vi "Cross_Moments.vi"(0 "U":dbl[](array[numeric]) format="%.2f", 1 "W":dbl[](array[numeric]) format="%.2f", 2 "Block No":i32=1, 3 "Inst names":string[](array[string]), 5 "Shift in":dbl[](array[numeric]) format="%.2f", 8 "Indicies":i32[](array[numeric])) -> (14 "Correlations Only":string[](array[string]), 15 "All Results for file":string[](array[string]), 17 "Velocity Cluster Array Out":T1[](array[typedef]) {"u^4" format="%.2f"; "Mean % Err" format="%.2f"; "u^4/(u^2)^2 -3" format="%.2f"; "u^3/(u^2)^(1.5)" format="%.2f"; "u^2" format="%.2f"; "% u'/U" format="%.2f"; "U" format="%.2f"}, 19 "Shift out":dbl[](array[numeric]) format="%.2f")   [LabVIEW 2010]
uses:
  Controls/Velocity_cluster.ctl
  Globals/Meas_global.vi
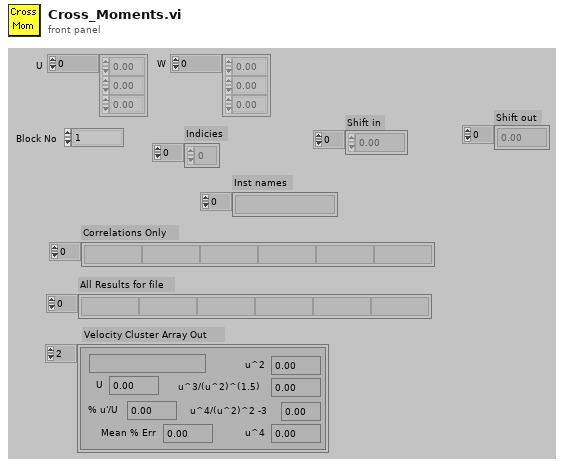
[diagram p1: front panel]
types:
  T1 = typedef "Velocity_cluster.ctl" = cluster{"Name":string, "U":dbl, "u^2":dbl, "u^3/(u^2)^(1.5)":dbl, "u^4/(u^2)^2 -3":dbl, "% u'/U":dbl, "Mean % Err":dbl, "u^4":dbl}
  T2 = typedef "Correlation_cluster.ctl" = cluster{"U inst":string, "W inst":string, "uw":dbl, "uw/u'w'":dbl, "u^2w":dbl, "uw^2":dbl, "uw^3":dbl, "u^3w":dbl, "u^2w^2":dbl}
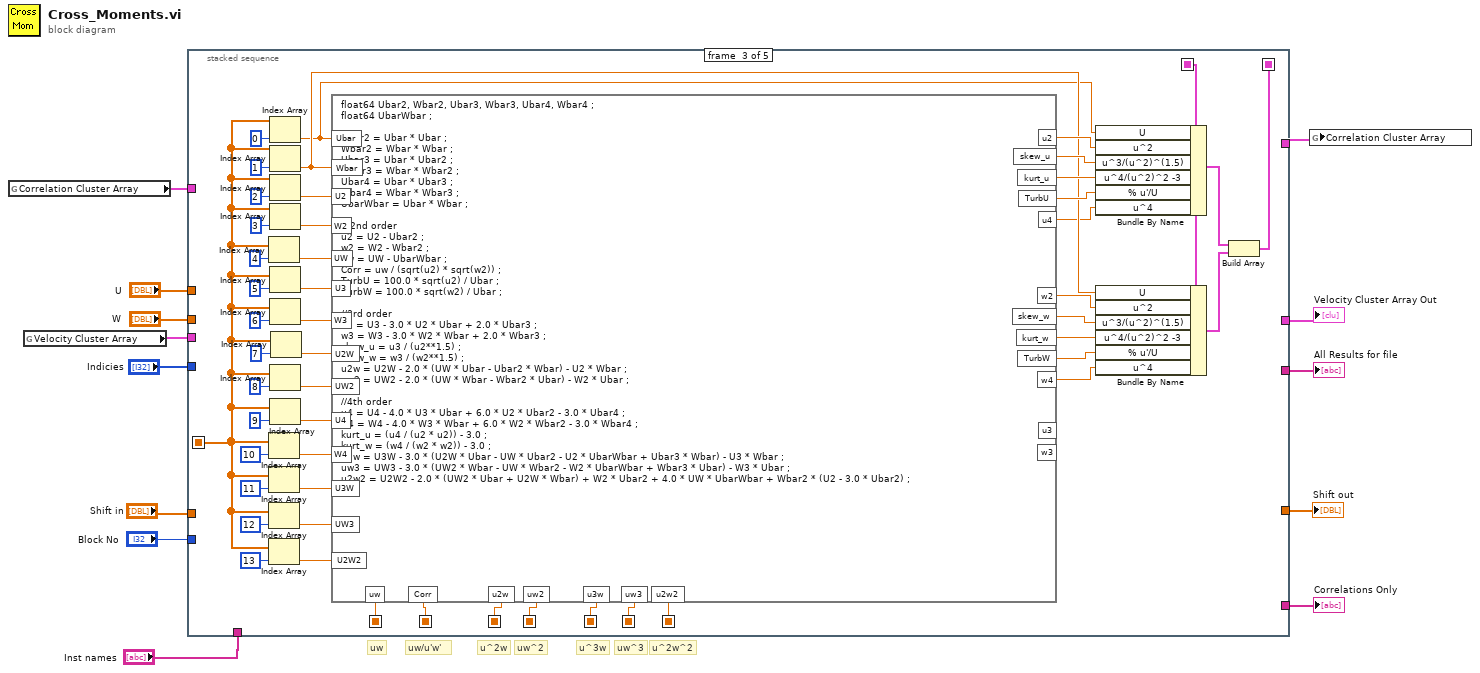
[diagram p0: block diagram]
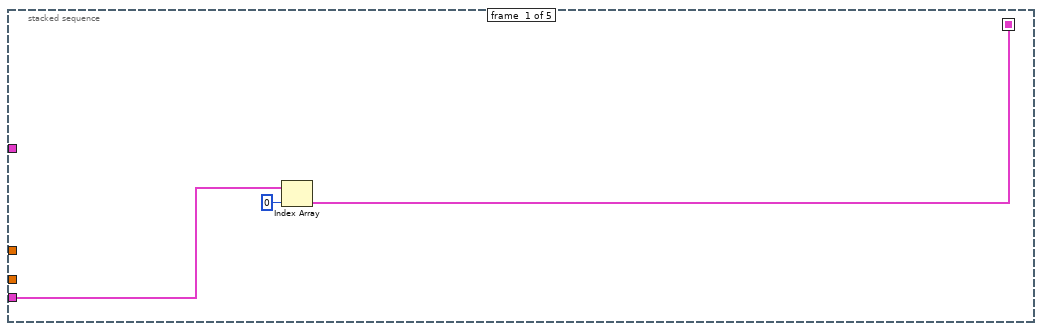
[diagram p2: hidden frame]
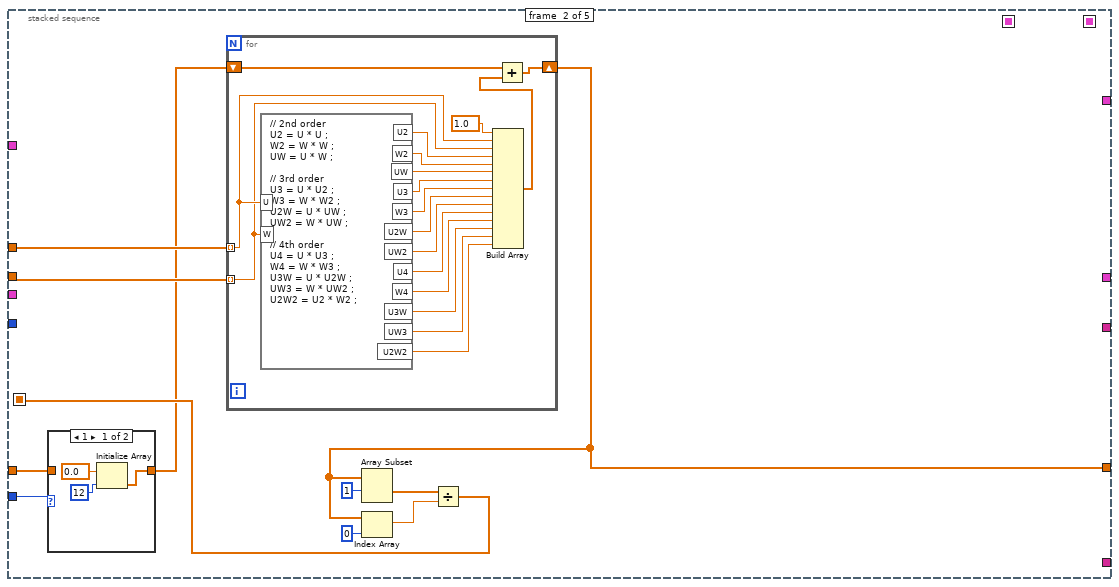
[diagram p3: hidden frame]
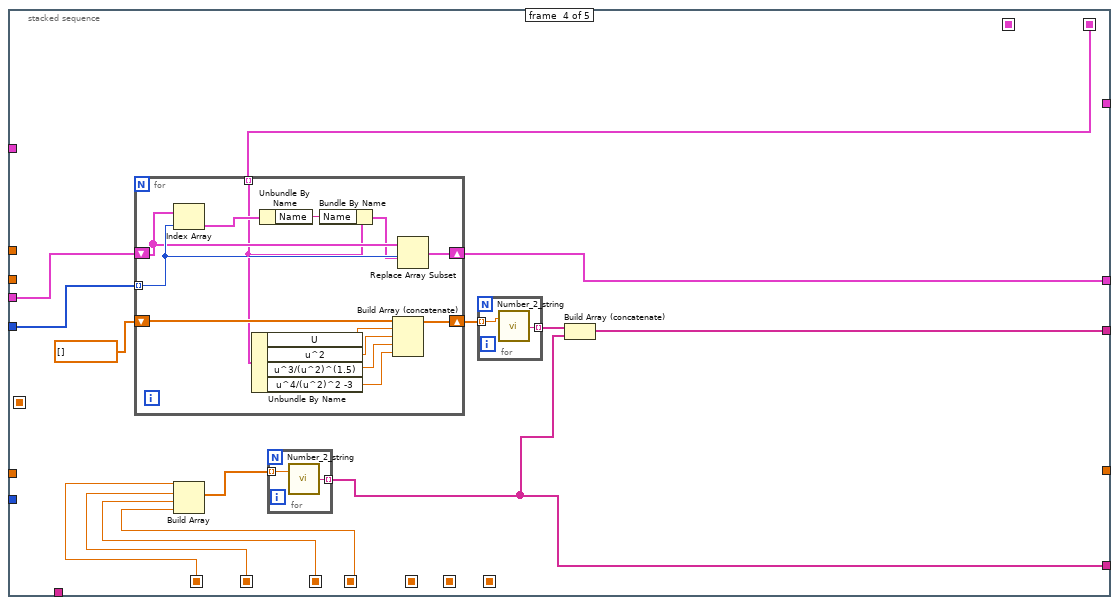
[diagram p5: hidden frame]
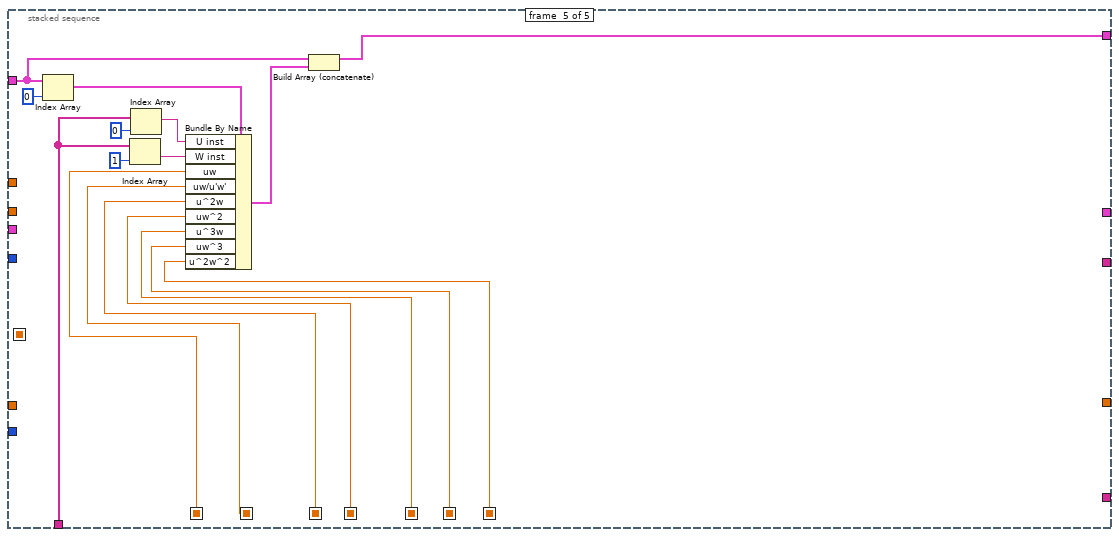
[diagram p6: hidden frame]
diagram:
  # "uw^2"
  # "u^2w"
  # "uw/u'w'"
  # "uw"
  # "u^2w^2"
  # "uw^3"
  # "u^3w"
  n1 = global read "Meas_global.vi" "Correlation Cluster Array"() -> (w10:T2[])
  n2 = global read "Meas_global.vi" "Velocity Cluster Array"() -> (w5:T1[])
  n3 = stacked-sequence {
    seq-local: [_ _ w91 _ _] -> [_ _ _ w113 w146]
    seq-local: [_ _ w90 _ _] -> [_ _ _ w112 w145]
    seq-local: [_ w20 _ _ _] -> [_ _ w56 _ _]
    seq-local: [_ _ w85 _ _] -> [_ _ _ w111 w135]
    seq-local: [_ _ w84 _ _] -> [_ _ _ w110 w134]
    seq-local: [w14 _ _ _ _] -> [_ _ w76 _ _]
    seq-local: [_ _ w65 _ _] -> [_ _ _ w106 _]
    seq-local: [_ _ w50 _ _] -> [_ _ _ _ w133]
    seq-local: [_ _ w51 _ _] -> [_ _ _ _ w132]
    seq-local: [_ _ w52 _ _] -> [_ _ _ _ w131]
    tunnel: "U" -> [_ w27 _ _ _]
    tunnel: [_ w21 _ _ _] -> w12
    tunnel: "Shift in" -> [_ w18 _ _ _]
    tunnel: [_ _ _ w100 _] -> w11
    tunnel: w10 -> [_ _ _ _ w143]
    tunnel: [_ _ _ _ w141] -> w9
    tunnel: "W" -> [_ w26 _ _ _]
    tunnel: "Inst names" -> [_ _ _ _ w138]
    tunnel: w5 -> [w15 _ _ w109 _]
    tunnel: [_ _ _ w108 _] -> w1
    tunnel: "Indicies" -> [_ _ _ w107 _]
    tunnel: [_ _ _ w104 _] -> w4
    tunnel: "Block No" -> [_ w19 _ _ _]
    frame #0 {
      n4 = Index Array(array=w15, index=0 ("Index")) -> (element=w14:T1)
    }
    frame #1 {
      n5 = case shown="1" w19 {
        tunnel: [w28 w31] -> w17
        tunnel: w18 -> [_ w31]
        frame 1 {
          n6 = Initialize Array(0.0 ("Element Data"), 12 ("Dimension Size")) -> (w28:dbl[])
        }
        frame 2, Default {
        }
      }
      n7 = for {
        shift-right: [w44] -> w21
        shift-left: w17 -> [w49]
        tunnel: w27 -> [w42] mode=indexing
        tunnel: w26 -> [w41] mode=indexing
        n8 = formula code="// 2nd order\nU2 = U * U ;\nW2 = W * W ;\nUW = U * W ;\n\n// 3rd order\nU3 = U * U2 ;\nW3 = W * W2 ;\nU2W = U * UW ;\nUW2 = W * UW ;\n\n// 4th order\nU4 = U * U3 ;\nW4 = W * W3 ;\nU3W = U * U2W ;\nUW3 = W * UW2 ;\nU2W2 = U2 * W2 ;"("W"=w41, "U"=w42) -> ("UW"=w45:dbl, "U2"=w47:dbl, "W2"=w46:dbl, "U2W"=w38:dbl, "UW2"=w37:dbl, "U3"=w40:dbl, "U4"=w36:dbl, "W3"=w39:dbl, "W4"=w35:dbl, "U3W"=w34:dbl, "UW3"=w33:dbl, "U2W2"=w32:dbl)
        n9 = Build Array(1.0 ("Input Element"), w42, w41, w47, w46, w45, w40, w39, w38, w37, w36, w35, w34, w33, w32) -> (w48:dbl[])
        n10 = Add(x=w49, y=w48) -> (x+y=w44:dbl[])
      }
      n11 = Array Subset(array=w21, index=1 ("Array Index")) -> (w23:dbl[])  [unwired: 1 in]
      n12 = Index Array(array=w21, index=0 ("Index")) -> (element=w22:dbl)
      n13 = Divide(x=w23, y=w22) -> (x/y=w20:dbl[])
    }
    frame #2 {
      n14 = Index Array(array=w56, index=4) -> (element=w92:dbl)
      n15 = Index Array(array=w56, index=10) -> (element=w79:dbl)
      n16 = Index Array(array=w56, index=11) -> (element=w53:dbl)
      n17 = Index Array(array=w56, index=12) -> (element=w54:dbl)
      n18 = Index Array(array=w56, index=13) -> (element=w55:dbl)
      n19 = Index Array(array=w56, index=0) -> (element=w63:dbl)
      n20 = Index Array(array=w56, index=1) -> (element=w64:dbl)
      n21 = Index Array(array=w56, index=2) -> (element=w94:dbl)
      n22 = Index Array(array=w56, index=3) -> (element=w93:dbl)
      n23 = Index Array(array=w56, index=5) -> (element=w87:dbl)
      n24 = Index Array(array=w56, index=6) -> (element=w86:dbl)
      n25 = Index Array(array=w56, index=8) -> (element=w77:dbl)
      n26 = Index Array(array=w56, index=9) -> (element=w80:dbl)
      n27 = Index Array(array=w56, index=7) -> (element=w78:dbl)
      n28 = formula code="float64 Ubar2, Wbar2, Ubar3, Wbar3, Ubar4, Wbar4 ;\nfloat64 UbarWbar ;\n\nUbar2 = Ubar * Ubar ;\nWbar2 = Wbar * Wbar ;\nUbar3 = Ubar * Ubar2 ;\nWbar3 = Wbar * Wbar2 ;\nUbar4 = Ubar * Ubar3 ;\nWbar4 = Wbar * Wbar3 ;\nUbarWbar = Ubar * Wbar ;\n\n// 2nd order\nu2 = U2 - Ubar2 ;\nw2 = W2 - Wbar2 ;\nuw = UW - UbarWbar ;\nCorr = uw / (sqrt(u2) * sqrt(w2)) ;\nTurbU = 100.0 * sqrt(u2) / Ubar ;\nTurbW = 100.0 * sqrt(w2) / Ubar ;\n\n//3rd order\nu3 = U3 - 3.0 * U2 * Ubar + 2.0 * Ubar3 ;\nw3 = W3 - 3.0 * W2 * Wbar + 2.0 * Wbar3 ;\nskew_u = u3 / (u2**1.5) ;\nskew_w = w3 / (w2**1.5) ;\nu2w = U2W - 2.0 * (UW * Ubar - Ubar2 * Wbar) - U2 * Wbar ;\nuw2 = UW2 - 2.0 * (UW * Wbar - Wbar2 * Ubar) - W2 * Ubar ;\n\n//4th order\nu4 = U4 - 4.0 * U3 * Ubar + 6.0 * U2 * Ubar2 - 3.0 * Ubar4 ;\nw4 = W4 - 4.0 * W3 * Wbar + 6.0 * W2 * Wbar2 - 3.0 * Wbar4 ;\nkurt_u = (u4 / (u2 * u2)) - 3.0 ;\nkurt_w = (w4 / (w2 * w2)) - 3.0 ;\nu3w = U3W - 3.0 * (U2W * Ubar - UW * Ubar2 - U2 * UbarWbar + Ubar3 * Wbar) - U3 * Wbar ;\nuw3 = UW3 - 3.0 * (UW2 * Wbar - UW * Wbar2 - W2 * UbarWbar + Wbar3 * Ubar) - W3 * Ubar ;\nu2w2 = U2W2 - 2.0 * (UW2 * Ubar + U2W * Wbar) + W2 * Ubar2 + 4.0 * UW * UbarWbar + Wbar2 * (U2 - 3.0 * Ubar2) ;"("Ubar"=w63, "Wbar"=w64, "W2"=w93, "UW"=w92, "U2"=w94, "U3"=w87, "W3"=w86, "U2W"=w78, "U4"=w80, "UW2"=w77, "W4"=w79, "U3W"=w53, "UW3"=w54, "U2W2"=w55) -> ("uw"=w91:dbl, "u2"=w68:dbl, "w2"=w74:dbl, "Corr"=w90:dbl, "u2w"=w85:dbl, "uw2"=w84:dbl, "skew_u"=w69:dbl, "kurt_u"=w70:dbl, "skew_w"=w73:dbl, "kurt_w"=w72:dbl, "TurbU"=w75:dbl, "TurbW"=w71:dbl, "u4"=w61:dbl, "w4"=w62:dbl, "u3w"=w50:dbl, "uw3"=w51:dbl, "u2w2"=w52:dbl)  [unwired: 2 out]
      n29 = Bundle By Name(cluster=w76, "U"=w63, "u^2"=w68, "u^3/(u^2)^(1.5)"=w69, "u^4/(u^2)^2 -3"=w70, "% u'/U"=w75, "u^4"=w61) -> (w66:T1)
      n30 = Bundle By Name(cluster=w76, "U"=w64, "u^2"=w74, "u^3/(u^2)^(1.5)"=w73, "u^4/(u^2)^2 -3"=w72, "% u'/U"=w71, "u^4"=w62) -> (w67:T1)
      n31 = Build Array(w66, w67) -> (w65:T1[])
    }
    frame #3 {
      n32 = for {
        shift-right: [w130] -> w108
        shift-left: w109 -> [w122]
        tunnel: w107 -> [w123] mode=indexing
        tunnel: w106 -> [w120] mode=indexing
        shift-right: [w128] -> w102
        shift-left: dbl[] [] -> [w129]
        n33 = Index Array(array=w122, index=w123) -> (element=w121:T1)
        n34 = Unbundle By Name(w120) -> ("U"=w127:dbl, "u^2"=w126:dbl, "u^3/(u^2)^(1.5)"=w125:dbl, "u^4/(u^2)^2 -3"=w124:dbl)
        n35 = Unbundle By Name(w121) -> ("Name"=w119:string)
        n36 = Bundle By Name(cluster=w120, "Name"=w119) -> (w118:T1)
        n37 = Build Array (concatenate)(w129, w127, w126, w125, w124) -> (w128:dbl[])
        n38 = Replace Array Subset(array=w122, new element=w118, index=w123) -> (w130:T1[])
      }
      n39 = Build Array(w113, w112, w111, w110) -> (w101:dbl[])
      n40 = for {
        tunnel: w101 -> [w115] mode=indexing
        tunnel: [w114] -> w100 mode=indexing
        n41 = call "Number_2_string.vi"("number"=w115) -> ("String"=w114:string)  [unwired: 1 in]
      }
      n42 = for {
        tunnel: [w117] -> w103 mode=indexing
        tunnel: w102 -> [w116] mode=indexing
        n43 = call "Number_2_string.vi"("number"=w116) -> ("String"=w117:string)  [unwired: 1 in]
      }
      n44 = Build Array (concatenate)(w103, w100) -> (w104:string[])
    }
    frame #4 {
      n45 = Index Array(array=w143, index=0) -> (element=w147:T2)
      n46 = Index Array(array=w138, index=1) -> (element=w136:string)
      n47 = Index Array(array=w138, index=0) -> (element=w137:string)
      n48 = Bundle By Name(cluster=w147, "U inst"=w137, "W inst"=w136, "uw"=w146, "uw/u'w'"=w145, "u^2w"=w135, "uw^2"=w134, "u^3w"=w133, "uw^3"=w132, "u^2w^2"=w131) -> (w142:T2)
      n49 = Build Array (concatenate)(w143, w142) -> (w141:T2[])
    }
  }
  "Shift out" <- w12
  "Correlations Only" <- w11
  "All Results for file" <- w4
  "Velocity Cluster Array Out" <- w1
  n50 = global write "Meas_global.vi" "Correlation Cluster Array"(w9) -> ()
